vi "Focus Initialize.vi"(8 "error in (no error)":errorcluster, 10 "Motion Settings":T1, 11 "NewFocus in":refnum<class "NewFocus.lvclass">) -> (0 "error out":errorcluster, 1 "Motor Positions":i32[](array[numeric]), 2 "Device Name":string, 3 "NewFocus out":refnum<class "NewFocus.lvclass">)   [LabVIEW 2024, in "NewFocus.lvclass"]
uses:
  NewFocus.lvclass
  C:/Development/Prime-RIMAS/Focus/Focus Class/Focus Class.lvclass
  Focus cluster Motion Settings.ctl
  NewFocus.lvclass/NewFocus.ctl
  Focus Class/Focus Class.lvclass/Focus Class.ctl
  Focus Class/Focus Class.lvclass
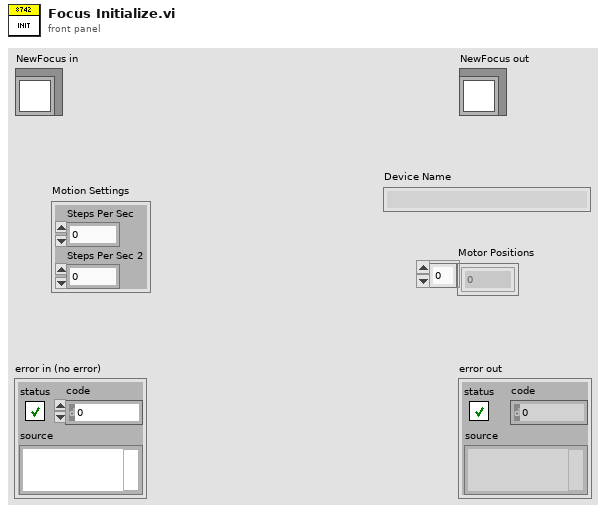
[diagram p1: front panel]
types:
  T1 = typedef "Focus cluster Motion Settings.ctl" = cluster{"Steps Per Sec":i32, "Steps Per Sec 2":i32}
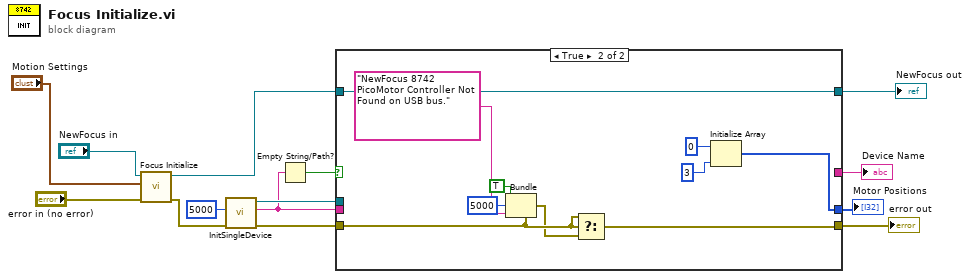
[diagram p0: block diagram]
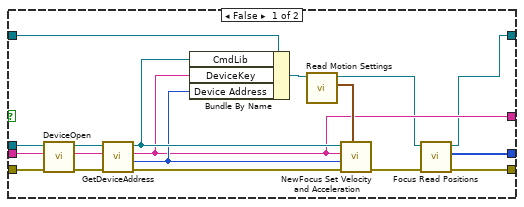
[diagram p2: hidden frame]
diagram:
  n1 = call-parent "Focus Initialize.vi"("error in (no error)"="error in (no error)", "Motion Settings"="Motion Settings", "Focus Class in"="NewFocus in") -> ("error out"=w12:errorcluster, "Focus Class out"=w7:refnum<class "NewFocus.lvclass">)  [unwired: 5 in, 2 out]
  n2 = call "InitSingleDevice.vi"("error in (no error)"=w12, "msecDelayForDiscovery"=5000) -> ("error out"=w10:errorcluster, "DeviceKey Out"=w4:string, "CmdLib Out"=w8:refnum<k24>)  [unwired: 3 in]
  n3 = Empty String/Path?(string/path=w4) -> (empty?=w9:bool)
  n4 = case shown="True" w9 {
    tunnel: w10 -> [w31 w40]
    tunnel: w8 -> [w30 _]
    tunnel: w7 -> [w32 w36]
    tunnel: [w18 w36] -> w6
    tunnel: [w16 w37] -> w5
    tunnel: w4 -> [w29 _]
    tunnel: [w20 _] -> w2
    tunnel: [w15 w33] -> w1
    frame False {
      n5 = call "DeviceOpen.vi"("error in (no error)"=w31, "DeviceKey In"=w29, "CmdLib In"=w30) -> ("error out"=w28:errorcluster, "DeviceKey Out"=w26:string, "CmdLib Out"=w27:refnum<k24>)  [unwired: 2 in]
      n6 = call "GetDeviceAddress.vi"("error in (no error)"=w28, "DeviceKey In"=w26, "CmdLib In"=w27) -> ("error out"=w25:errorcluster, "Device Address"=w21:i32, "DeviceKey Out"=w20:string, "CmdLib Out"=w22:refnum<k24>)  [unwired: 5 in]
      n7 = Bundle By Name(cluster=w32, "CmdLib"=w22, "DeviceKey"=w20, "Device Address"=w21) -> (w24:refnum<class "NewFocus.lvclass">)
      n8 = call "Read Motion Settings.vi"("Focus Class in"=w24) -> ("Motion Settings"=w23:T1, "Focus Class out"=w19:refnum<class "NewFocus.lvclass">)  [unwired: 8 in, 1 out]
      n9 = call "NewFocus Set Velocity and Acceleration.vi"("Motion Settings"=w23, "error in (no error)"=w25, "Device Address In"=w21, "DeviceKey In"=w20, "CmdLib In"=w22) -> ("error out"=w17:errorcluster)  [unwired: 6 in]
      n10 = call-dynamic "Focus Read Positions.vi"("error in (no error)"=w17, "NewFocus in"=w19) -> ("error out"=w16:errorcluster, "Motor Positions"=w15:i32[], "NewFocus out"=w18:refnum<class "NewFocus.lvclass">)  [unwired: 7 in]
    }
    frame True {
      n11 = Bundle(cluster=w40, "status"=TRUE, "code"=5000, "source"="NewFocus 8742 PicoMotor Controller Not Found on USB bus.") -> (w39:errorcluster)
      n12 = Select(t=w40, s=w40, f=w39) -> (s? t:f=w37:errorcluster)
      n13 = Initialize Array(0, 3) -> (w33:i32[])
    }
  }
  "error out" <- w5
  "NewFocus out" <- w6
  "Device Name" <- w2
  "Motor Positions" <- w1
